vi "Kill.vi"() -> ()   [LabVIEW 2011]
panel:
  in  "Kill":bool
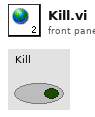
[diagram p1: front panel]
diagram:
